vi "Tick Count.vi"() -> ()   [LabVIEW 2023]
panel:
  out "Tick Count":u64
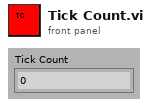
[diagram p1: front panel]
diagram:
